vi "set_voltage.vi"(8 "error in":errorcluster, 10 "voltage":dbl, 11 "VISA resource name":refnum<visa-resource-name>="COM1") -> (0 "error out":errorcluster, 3 "Response":string)   [LabVIEW 2020]
panel:
  out "command":string
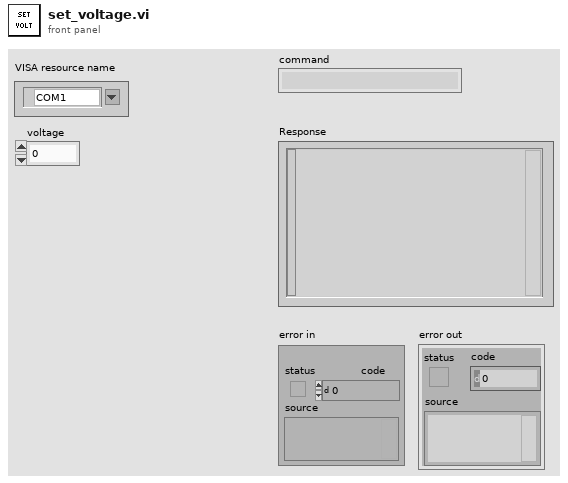
[diagram p1: front panel]
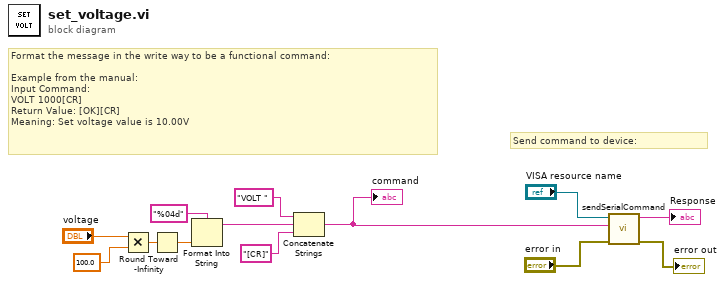
[diagram p0: block diagram]
diagram:
  # "Send command to device:"
  # "Format the message in the write way to be a functional command:\n\nExample from the manual:\nInput Command:\nVOLT 1000[CR]\nReturn Value: [OK][CR]\nMeaning: Set voltage value is 10.00V"
  n1 = Multiply(x="voltage", y=100.0) -> (x*y=w10:dbl)
  n2 = Round Toward -Infinity(1:w10) -> (0:w7:dbl)
  n3 = Format Into String(format string="%04d", w7) -> (resulting string=w8:string)  [unwired: 2 in, 1 out]
  n4 = Concatenate Strings("VOLT " ("string"), w8, "[CR]" ("string")) -> (w2:string)
  "command" <- w2
  n5 = call "sendSerialCommand.vi"("error in (no error)"="error in", "Command"=w2, "VISA resource name"="VISA resource name") -> ("error out"=→"error out":errorcluster, "Response"=→"Response":string)  [unwired: 7 in]
